vi "GSP_Parser.vi"(5 "Queue F2":refnum<queue>, 6 "Queue F1":refnum<queue>, 7 "Command":string) -> (3 "Reply":string)   [LabVIEW 2015]
uses:
  SystemUtil/Command.ctl
  Primary Filter/GSP_F1_Global.vi
  Secondary Filter/GSP_F2_Global.vi
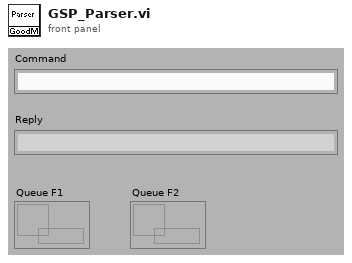
[diagram p1: front panel]
types:
  T1 = typedef "Command.ctl" = cluster{"Command":string, "Parameter":string}
  T2 = typedef "ThreadStates.ctl" = enum16{"Waiting", "Scripting", "Uninitialized", "Error"}
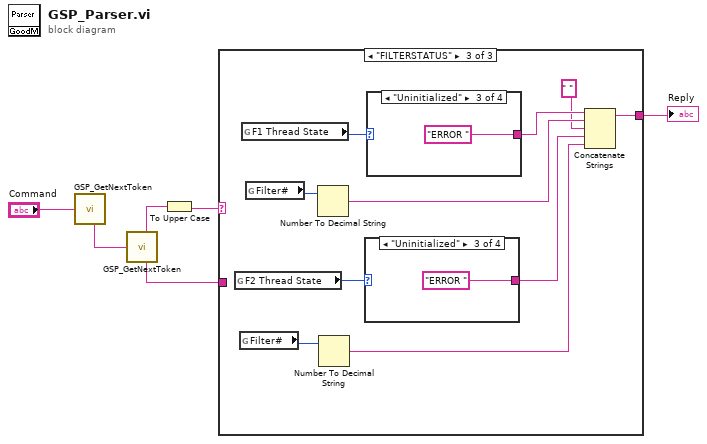
[diagram p0: block diagram]
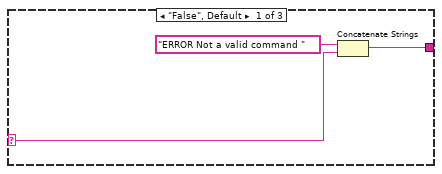
[diagram p2: hidden frame]
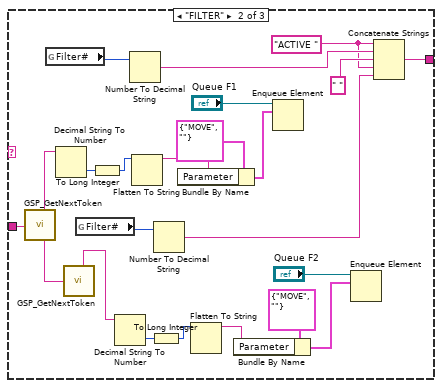
[diagram p3: hidden frame]
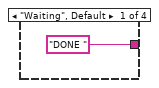
[diagram p4: hidden frame]
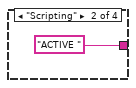
[diagram p5: hidden frame]
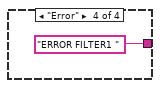
[diagram p6: hidden frame]
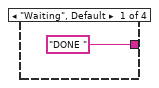
[diagram p7: hidden frame]
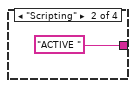
[diagram p8: hidden frame]
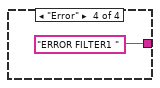
[diagram p9: hidden frame]
diagram:
  n1 = call "GSP_GetNextToken.vi"("Input string"="Command") -> ("Output string"=w5:string)  [unwired: 4 in, 1 out]
  n2 = call "GSP_GetNextToken.vi"("Input string"=w5) -> ("Token"=w4:string, "Output string"=w2:string)  [unwired: 4 in]
  n3 = To Upper Case(1:w4) -> (0:w3:string)
  n4 = case shown="\"FILTERSTATUS\"" w3 {
    selector: w3 -> [w7 _ _]
    tunnel: w2 -> [_ w32 _]
    tunnel: [w8 w23 w40] -> w1
    frame "False", Default {
      n5 = Concatenate Strings("ERROR Not a valid command ", w7) -> (w8:string)
    }
    frame "FILTER" {
      w12 = "ACTIVE "
      n6 = call "GSP_GetNextToken.vi"("Input string"=w32) -> ("Token"=w25:string, "Output string"=w14:string)  [unwired: 4 in]
      n7 = global read "GSP_F1_Global.vi" "Filter#"() -> (w22:i32)
      n8 = Decimal String To Number(string=w25) -> (number=w30:i32)  [unwired: 2 in, 1 out]
      n9 = call "GSP_GetNextToken.vi"("Input string"=w14) -> ("Token"=w10:string)  [unwired: 4 in, 1 out]
      n10 = global read "GSP_F2_Global.vi" "Filter#"() -> (w13:i32)
      n11 = To Long Integer(number=w30) -> (32bit integer=w31:i32)
      n12 = Decimal String To Number(string=w10) -> (number=w17:i32)  [unwired: 2 in, 1 out]
      n13 = Number To Decimal String(number=w22) -> (decimal integer string=w21:string)  [unwired: 1 in]
      n14 = Flatten To String(anything=w31) -> (data string=w27:string)  [unwired: 3 in, 2 out]
      n15 = To Long Integer(number=w17) -> (32bit integer=w16:i32)
      n16 = Number To Decimal String(number=w13) -> (decimal integer string=w11:string)  [unwired: 1 in]
      n17 = Bundle By Name(cluster=T1 {"Command"="MOVE", "Parameter"=""} ("element"), "Parameter"=w27) -> (w26:T1)
      n18 = Flatten To String(anything=w16) -> (data string=w15:string)  [unwired: 3 in, 2 out]
      n19 = Bundle By Name(cluster=T1 {"Command"="MOVE", "Parameter"=""} ("element"), "Parameter"=w15) -> (w18:T1)
      n20 = Enqueue Element(queue="Queue F1", element=w26) -> ()  [unwired: 2 in, 3 out]
      n21 = Enqueue Element(queue="Queue F2", element=w18) -> ()  [unwired: 2 in, 3 out]
      n22 = Concatenate Strings(w12, w21, " ", w12, w11) -> (w23:string)
    }
    frame "FILTERSTATUS" {
      n23 = global read "GSP_F2_Global.vi" "F2 Thread State"() -> (w33:T2)
      n24 = global read "GSP_F2_Global.vi" "Filter#"() -> (w36:i32)
      n25 = global read "GSP_F1_Global.vi" "F1 Thread State"() -> (w39:T2)
      n26 = global read "GSP_F1_Global.vi" "Filter#"() -> (w42:i32)
      n27 = Number To Decimal String(number=w42) -> (decimal integer string=w38:string)  [unwired: 1 in]
      n28 = Number To Decimal String(number=w36) -> (decimal integer string=w34:string)  [unwired: 1 in]
      n29 = case shown="\"Uninitialized\"" w33 {
        tunnel: ["DONE " "ACTIVE " "ERROR " "ERROR FILTER1 "] -> w35
        frame "Waiting", Default {
        }
        frame "Scripting" {
        }
        frame "Uninitialized" {
        }
        frame "Error" {
        }
      }
      n30 = case shown="\"Uninitialized\"" w39 {
        tunnel: ["DONE " "ACTIVE " "ERROR " "ERROR FILTER1 "] -> w41
        frame "Waiting", Default {
        }
        frame "Scripting" {
        }
        frame "Uninitialized" {
        }
        frame "Error" {
        }
      }
      n31 = Concatenate Strings(w41, w38, " ", w35, w34) -> (w40:string)
    }
  }
  "Reply" <- w1
